vi "read.vi"(7 "timeout (ms)":i32, 8 "error in (no error)":errorcluster, 9 "number of channels":i32, 10 "block size":i32, 11 "FPGAWrapperRK110909Throughput in":refnum<class "FPGAWrapperRK110909Throughput.lvclass">) -> (0 "error out":errorcluster, 1 "channels raw data block":T1, 2 "FIFO full?":bool, 3 "FPGAWrapperRK110909Throughput out":refnum<class "FPGAWrapperRK110909Throughput.lvclass">, 4 "timed out?":bool)   [LabVIEW 2010, in "FPGAWrapperRK110909Throughput.lvclass"]
uses:
  FPGAWrapperRK110909Throughput.lvclass
  GenericFPGAWrapper/GenericFPGAWrapper/GenericFPGAWrapper.lvclass
  <vilib>/Utility/error.llb/Error Cluster From Error Code.vi
  <vilib>/rvi/errors/niLvFpgaWhatHappensToTopLevelVI.ctl
  <vilib>/rvi/interface/common/niFpgaNodeNameForErrorReporting.ctl
  <vilib>/rvi/errors/niLvFpgaAdjustHostInterfaceError.vi
  <vilib>/rvi/interface/nirviReadWriteControl/nirviReadWriteControl.xnode
  NiFpgaLv.dll
  <vilib>/rvi/interface/nirviMethod/nirviMethod.xnode
  FPGA_reference.ctl
  common/arrays/pixel_raw_data_array.ctl
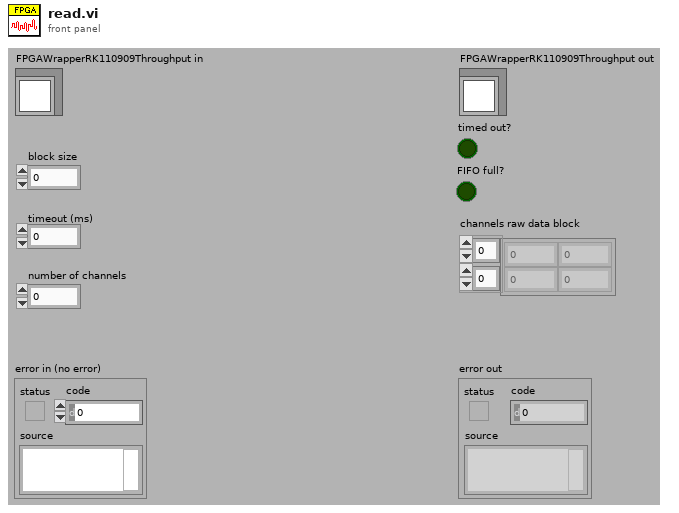
[diagram p1: front panel]
types:
  T1 = typedef "pixel_raw_data_array.ctl" = dbl[][]
  T2 = typedef "niFpgaNodeNameForErrorReporting.ctl" = enum16{"Open FPGA VI Reference", "Read/Write Control", "Invoke Method: Abort", "Invoke Method: Acknowledge IRQ", "Invoke Method: Download", "Invoke Method: FIFO.Configure", "Invoke Method: FIFO.Read", "Invoke Method: FIFO.Start", "Invoke Method: FIFO.Stop", "Invoke Method: FIFO.Write", "Invoke Method: Reset", "Invoke Method: Run", "Invoke Method: Wait on IRQ", "Close FPGA VI Reference"}
  T3 = typedef "niLvFpgaWhatHappensToTopLevelVI.ctl" = enum16{"top level VI scripted behind XNode", "top level VI inlined behind XNode"}
  T4 = typedef "FPGAWrapperRK110909Throughput.lvclass/FPGA_reference.ctl" = refnum<k20>
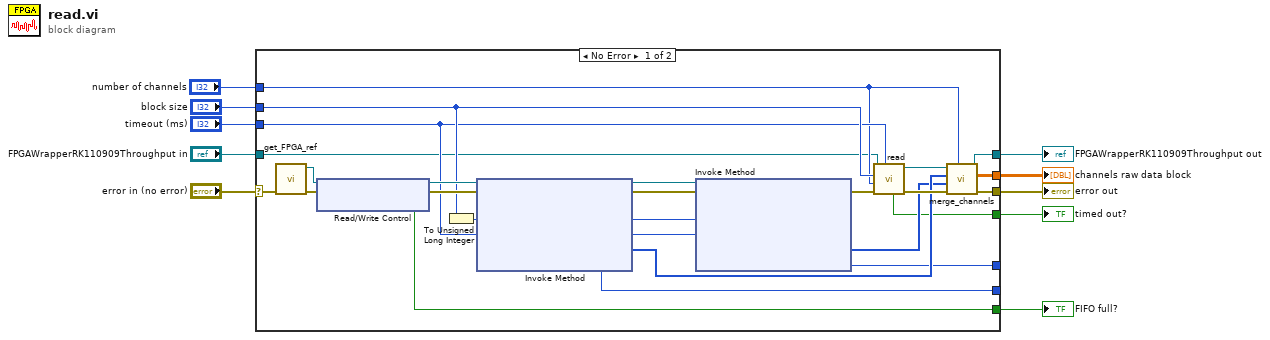
[diagram p0: block diagram]
diagram:
  n1 = case shown="No Error" "error in (no error)" {
    selector: "error in (no error)" -> [w15 w225]
    tunnel: "FPGAWrapperRK110909Throughput in" -> [w16 w224]
    tunnel: [w34 _] -> w2
    tunnel: "timeout (ms)" -> [w26 _]
    tunnel: "block size" -> [w27 _]
    tunnel: "number of channels" -> [w21 _]
    tunnel: [w11 w225] -> w5
    tunnel: [w20 _] -> w4
    tunnel: [w19 _] -> w3
    tunnel: [w18 _] -> _
    tunnel: [w17 _] -> _
    tunnel: [w12 _] -> w1
    frame No Error {
      n2 = call "get_FPGA_ref.vi"("error in"=w15) -> ("error out"=w14:errorcluster, "FPGA Reference"=w13:T4)  [unwired: 8 in, 1 out]
      n3 = xnode "Read/Write Control"("FPGA VI Reference In"=w13, "error in"=w14) -> ("FPGA VI Reference Out"=w32:T4, "error out"=w33:errorcluster, "FIFO overflow out"=w34:bool)
      n4 = To Unsigned Long Integer(number=w27) -> (unsigned 32bit integer=w28:u32)
      n5 = xnode "Invoke Method"("FPGA VI Reference In"=w32, "error in"=w33, "Number of Elements"=w28, "Timeout (ms)"=w26) -> ("FPGA VI Reference Out"=w31:T4, "error out"=w30:errorcluster, "Data"=w23:u16[], "Elements Remaining"=w17:u32)
      n6 = xnode "Invoke Method"("FPGA VI Reference In"=w31, "error in"=w30, "Number of Elements"=w28, "Timeout (ms)"=w26) -> ("error out"=w29:errorcluster, "Data"=w22:u16[], "Elements Remaining"=w18:u32)  [unwired: 1 out]
      n7 = call-parent "read.vi"("timeout (ms)"=w26, "error in (no error)"=w29, "number of channels"=w21, "block size"=w27, "GenericFPGAWrapper in"=w16) -> ("error out"=w25:errorcluster, "FIFO full?"=w19:bool, "GenericFPGAWrapper out"=w24:refnum<class "FPGAWrapperRK110909Throughput.lvclass">)  [unwired: 2 in, 2 out]
      n8 = call "merge_channels.vi"("number of channels"=w21, "error in (no error)"=w25, "FIFO_2"=w22, "FIFO_1"=w23, "FPGAWrapperRK110909Throughput.lvclass in"=w24) -> ("error out"=w11:errorcluster, "channels raw data block"=w20:T1, "FPGAWrapperRK110909Throughput.lvclass"=w12:refnum<class "FPGAWrapperRK110909Throughput.lvclass">)  [unwired: 4 in]
    }
    frame Error {
    }
  }
  "error out" <- w5
  "FPGAWrapperRK110909Throughput out" <- w1
  "FIFO full?" <- w2
  "channels raw data block" <- w4
  "timed out?" <- w3
